vi "InArea.vi"(8 "error in (no error)":errorcluster, 10 "Area in":T1, 11 "Coords":T2) -> (0 "error out":errorcluster, 1 "InArea":bool, 2 "Area out":T1)   [LabVIEW 2021, in "Menu.lvlib" / "Menu.lvclass"]
uses:
  Menu.lvclass
  <vilib>/Utility/miscctls.llb/LVPoint32TypeDef.ctl
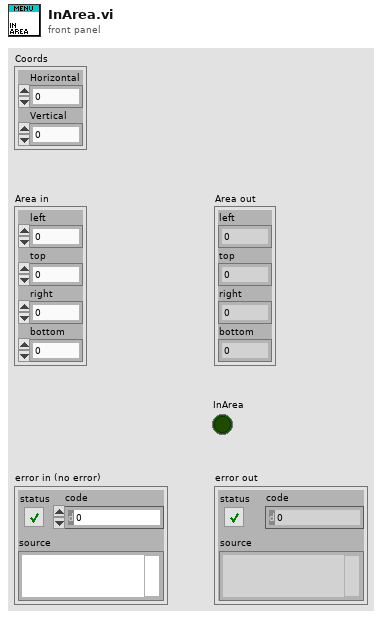
[diagram p1: front panel]
types:
  T1 = cluster{"left":i16, "top":i16, "right":i16, "bottom":i16}
  T2 = typedef "LVPoint32TypeDef.ctl" = cluster{"Horizontal":i32, "Vertical":i32}
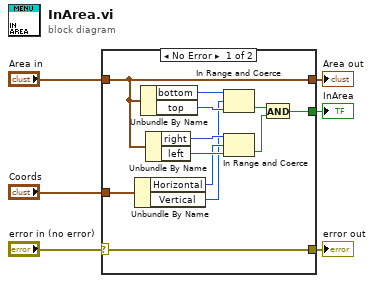
[diagram p0: block diagram]
diagram:
  n1 = case shown="No Error" "error in (no error)" {
    selector: "error in (no error)" -> [w8 w19]
    tunnel: "Coords" -> [w16 _]
    tunnel: "Area in" -> [w7 w20]
    tunnel: [w9 _] -> w4
    tunnel: [w8 w19] -> w2
    tunnel: [w7 w20] -> w1
    frame No Error {
      n2 = Unbundle By Name(w16) -> ("Horizontal"=w15:i32, "Vertical"=w12:i32)
      n3 = Unbundle By Name(w7) -> ("bottom"=w14:i16, "top"=w13:i16)
      n4 = Unbundle By Name(w7) -> ("right"=w18:i16, "left"=w17:i16)
      n5 = In Range and Coerce(upper limit=w14, x=w12, lower limit=w13) -> (In Range?=w10:bool)  [unwired: 1 out]
      n6 = In Range and Coerce(upper limit=w18, x=w15, lower limit=w17) -> (In Range?=w11:bool)  [unwired: 1 out]
      n7 = And(x=w10, y=w11) -> (x .and. y?=w9:bool)
    }
    frame Error {
    }
  }
  "Area out" <- w1
  "InArea" <- w4
  "error out" <- w2
